vi "postScanHoldtime.vi"(8 "error in (no error)":errorcluster, 11 "ChirpWave in":refnum<class "ChirpWave.lvclass">) -> (0 "error out":errorcluster, 1 "PostScanHoldTime":dbl[unit], 2 "PostscanHold?":bool=TRUE, 3 "ChirpWave out":refnum<class "ChirpWave.lvclass">)   [LabVIEW 2015, in "ChirpWave.lvclass"]
uses:
  ChirpWave.lvclass
  ChirpWave.lvclass/ChirpWave.ctl
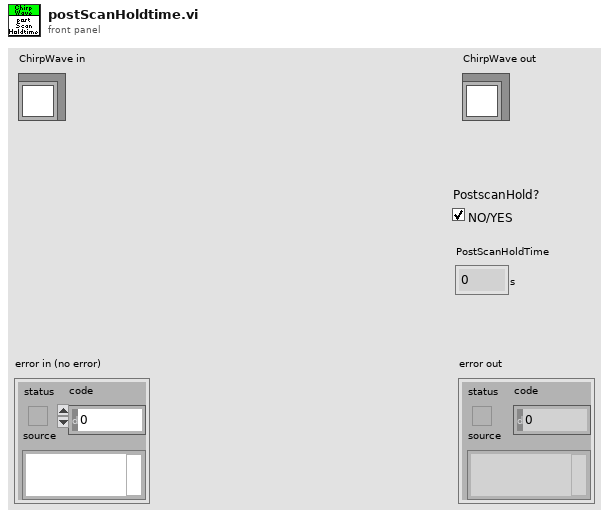
[diagram p1: front panel]
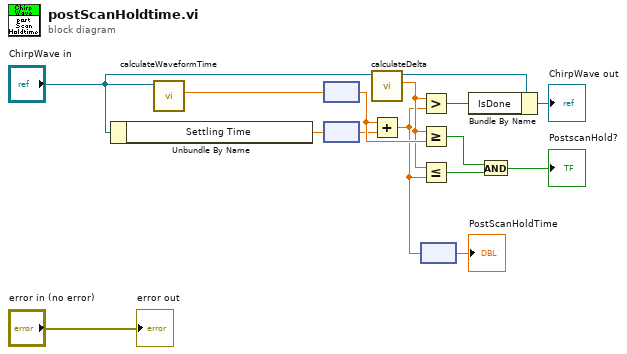
[diagram p0: block diagram]
diagram:
  n1 = Unbundle By Name("ChirpWave in") -> ("Settling Time"=w12:dbl[unit])
  n2 = call "calculateWaveformTime.vi"("ChirpWave in"="ChirpWave in") -> ("Waveform Time"=w14:dbl[unit])  [unwired: 8 in, 2 out]
  n3 = node(w14) -> (w13:dbl)
  n4 = node(w12) -> (w11:dbl)
  n5 = call "calculateDelta.vi"("ChirpWave in"="ChirpWave in") -> ("Delta Timestamp"=w7:dbl, "ChirpWave out"=w3:refnum<class "ChirpWave.lvclass">)  [unwired: 8 in, 1 out]
  n6 = Add(x=w13, y=w11) -> (x+y=w2:dbl)
  n7 = Greater?(x=w7, y=w2) -> (0:w6:bool)
  n8 = Greater Or Equal?(x=w7, y=w13) -> (x >= y?=w10:bool)
  n9 = Less Or Equal?(x=w7, y=w2) -> (x <= y?=w9:bool)
  n10 = node(w2) -> (→"PostScanHoldTime":dbl[unit])
  n11 = Bundle By Name(cluster=w3, "IsDone"=w6) -> (→"ChirpWave out":refnum<class "ChirpWave.lvclass">)
  n12 = And(x=w10, y=w9) -> (x .and. y?=→"PostscanHold?":bool)
  "error out" <- "error in (no error)"
